vi "Update data (SubVI).vi"(0 "Refnum in":T1, 1 "Kolom Username":string, 2 "Nilai User":string, 3 "Nama Table":string, 5 "Set Kolom":string, 9 "Set Nilai":string, 11 "error in (no error)":errorcluster, 12 "Kolom Role":string, 14 "Nilai Role":string) -> (4 "Refnum out":T1, 6 "Hasil Query":string, 15 "error out":errorcluster)   [LabVIEW 2025]
uses:
  <vilib>/addons/database/Connection.llb/Conn ObjectReference.ctl
  <vilib>/addons/database/Connection.llb/Conn Execute.vi
  <vilib>/addons/database/NI_Database_API.lvlib
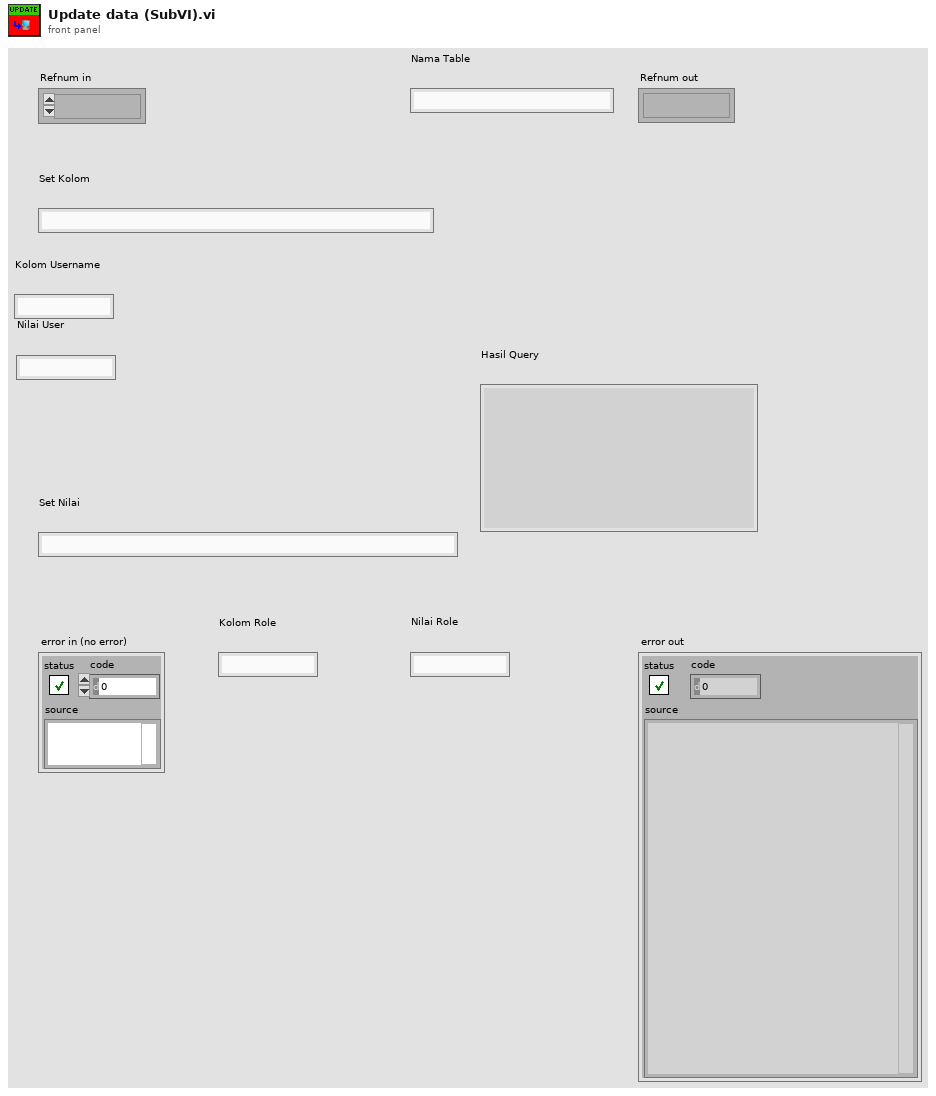
[diagram p1: front panel]
types:
  T1 = typedef "NI_Database_API.lvlib/Conn ObjectReference.ctl" = refnum<k1>
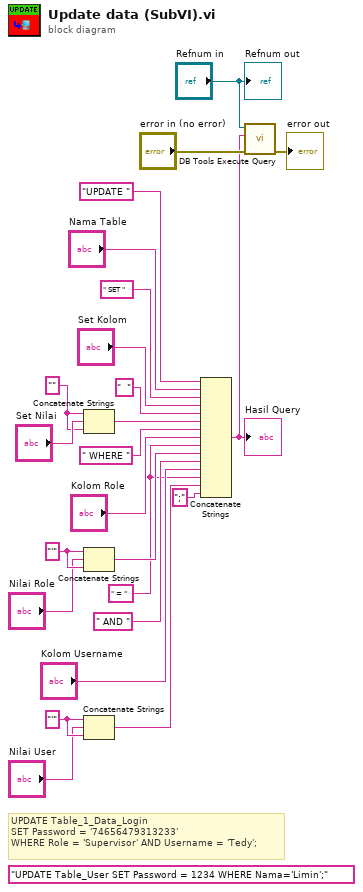
[diagram p0: block diagram]
diagram:
  w4 = "'" ("string")
  w10 = "'" ("string")
  w11 = "" ("string")
  w5 = " = " ("string")
  (unwired) "UPDATE Table_User SET Password = 1234 WHERE Nama='Limin';" ("SQL query")
  # "UPDATE Table_1_Data_Login\nSET Password = '74656479313233'\nWHERE Role = 'Supervisor' AND Username = 'Tedy';"
  n1 = Concatenate Strings(w11, "Set Nilai", w11) -> (w13:string)
  n2 = Concatenate Strings(w10, "Nilai Role", w10) -> (w8:string)
  n3 = Concatenate Strings(w4, "Nilai User", w4) -> (w2:string)
  n4 = Concatenate Strings("UPDATE " ("string"), "Nama Table", " SET " ("string"), "Set Kolom", "  " ("string"), w13, " WHERE " ("string"), "Kolom Role", w5, w8, " AND " ("string"), "Kolom Username", w5, w2, ";" ("string")) -> (w21:string)
  "Hasil Query" <- w21
  n5 = call-poly <vilib>:"DB Tools Execute Query.vi"("error in (no error)"="error in (no error)", "SQL query"=w21, "connection reference"="Refnum in") -> ("error out"=→"error out":errorcluster)  [unwired: 5 in, 1 out]
  "Refnum out" <- "Refnum in"
